vi "Read configuration.vi"(8 "error in":errorcluster, 11 "Polynomial Scale editor node in":refnum<class "Polynomial Scale editor node.lvclass">) -> (0 "error out":errorcluster, 2 "configuration":refnum<class "NISE_CEF_serializable configuration.lvclass">, 3 "Polynomial Scale editor node out":refnum<class "Polynomial Scale editor node.lvclass">)   [LabVIEW 2013, in "Polynomial Scale editor node.lvclass"]
uses:
  Polynomial Scale editor node.lvclass
  <vilib>/NI/Configuration Framework/serializable configuration/NISE_CEF_serializable configuration.lvclass
  Polynomial Scale editor node.lvclass/Polynomial Scale editor node.ctl
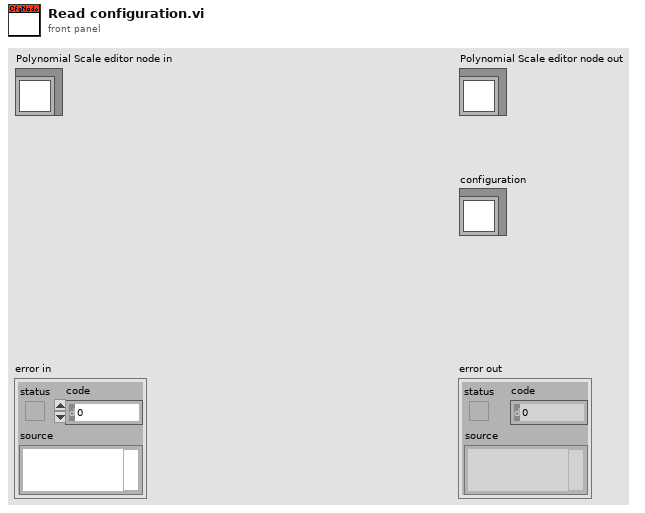
[diagram p1: front panel]
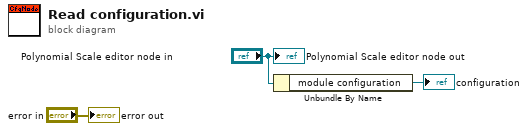
[diagram p0: block diagram]
diagram:
  n1 = Unbundle By Name("Polynomial Scale editor node in") -> ("module configuration"=→"configuration":refnum<class "Polynomial Scale configuration.lvclass">)
  "error out" <- "error in"
  "Polynomial Scale editor node out" <- "Polynomial Scale editor node in"
